vi "Unregister Logger by Name.vi"(8 "error in (no error)":errorcluster, 11 "name":string) -> (0 "error out":errorcluster, 3 "failure info":T1 {"Log Record"."timestamp" format="%<%x %.3X>T"})   [LabVIEW 2018, in "GLog.lvlib"]
uses:
  GLog.lvlib
  Failure Information.ctl
  Log Record.ctl
  logger_class/Internal Log Levels.ctl
  registry/Registry.lvlib
  logger_class/Logger.lvclass
panel:
  # "Connector Pane"
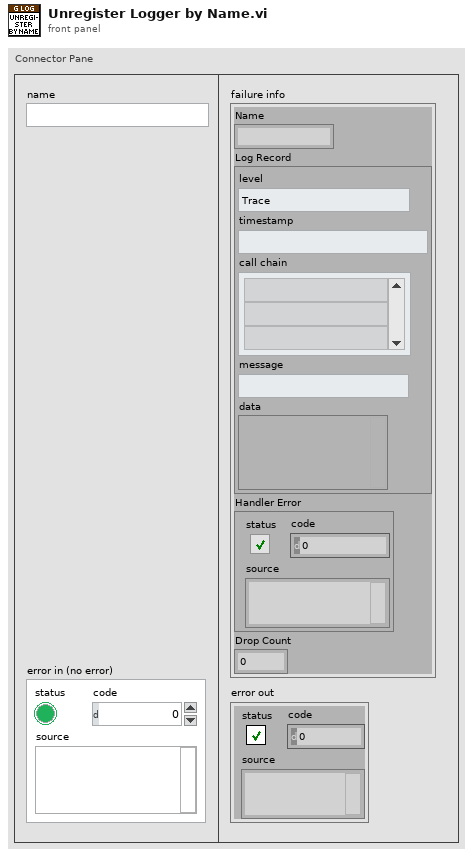
[diagram p1: front panel]
types:
  T1 = typedef "GLog.lvlib/Failure Information.ctl" = cluster{"Name":string, "Log Record":T2, "Handler Error":errorcluster, "Drop Count":u32}
  T2 = typedef "GLog.lvlib/Log Record.ctl" = cluster{"level":T3, "timestamp":timestamp, "call chain":string[], "message":string, "data":variant}
  T3 = typedef "GLog.lvlib/Internal Log Levels.ctl" = enum16{"Trace", "Debug", "Info", "Warning", "Error", "Critical", "Internal"}
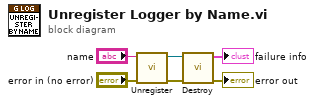
[diagram p0: block diagram]
diagram:
  n1 = call "Unregister.vi"("error in (no error)"="error in (no error)", "logger name"="name") -> ("error out"=w6:errorcluster, "logger"=w5:refnum<class "Logger.lvclass">)  [unwired: 8 in]
  n2 = call "Destroy.vi"("error in (no error)"=w6, "logger in"=w5) -> ("error out"=→"error out":errorcluster, "failure info"=→"failure info":T1)  [unwired: 8 in]
